vi "LossyAddToGrid.vi"(8 "error in (no error)":errorcluster, 9 "Coordinate":cluster{"x":i16, "y":i16}, 10 "Tilecode":u32, 11 "SnakeGame in":refnum<class "SnakeGame.lvclass">) -> (0 "error out":errorcluster, 3 "SnakeGame out":refnum<class "SnakeGame.lvclass">)   [LabVIEW 2019, in "RT_Game.lvlib" / "SnakeGame.lvclass"]
uses:
  SnakeGame.lvclass
  SnakeGame.lvclass/SnakeGame.ctl
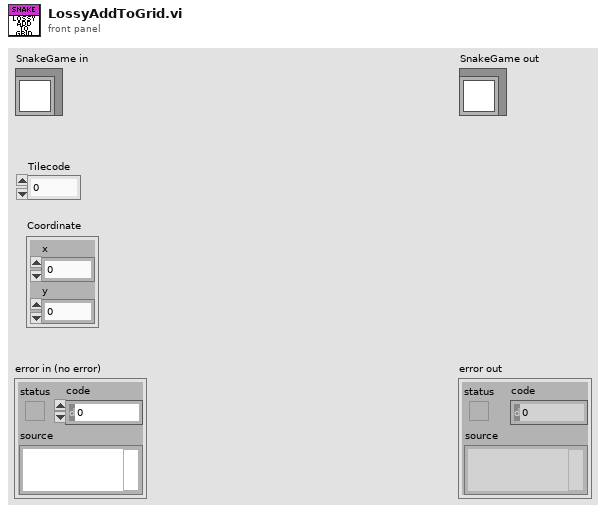
[diagram p1: front panel]
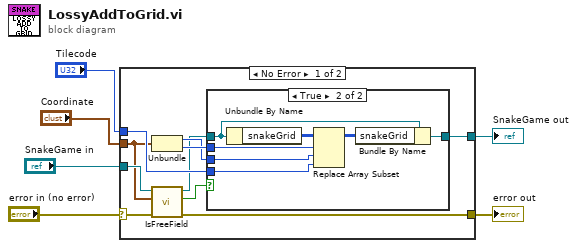
[diagram p0: block diagram]
diagram:
  n1 = case shown="No Error" "error in (no error)" {
    selector: "error in (no error)" -> [w10 w26]
    tunnel: [w9 w26] -> w5
    tunnel: [w16 w25] -> w3
    tunnel: "SnakeGame in" -> [w12 w25]
    tunnel: "Coordinate" -> [w8 _]
    tunnel: "Tilecode" -> [w15 _]
    frame No Error {
      n2 = Unbundle(w8) -> ("x"=w13:i16, "y"=w14:i16)
      n3 = call "IsFreeField.vi"("error in (no error)"=w10, "Coordinate"=w8, "SnakeGame in"=w12) -> ("error out"=w9:errorcluster, "Free?"=w7:bool, "SnakeGame out"=w11:refnum<class "SnakeGame.lvclass">)  [unwired: 6 in]
      n4 = case shown="True" w7 {
        tunnel: [w17 w24] -> w16
        tunnel: w15 -> [_ w22]
        tunnel: w14 -> [_ w21]
        tunnel: w13 -> [_ w20]
        tunnel: w11 -> [w17 w18]
        frame False {
        }
        frame True {
          n5 = Unbundle By Name(w18) -> ("snakeGrid"=w19:u32[][])
          n6 = Replace Array Subset(array=w19, new element=w22, index (row)=w21, index (col)=w20) -> (w23:u32[][])
          n7 = Bundle By Name(cluster=w18, "snakeGrid"=w23) -> (w24:refnum<class "SnakeGame.lvclass">)
        }
      }
    }
    frame Error {
    }
  }
  "error out" <- w5
  "SnakeGame out" <- w3
